vi "2dArrayTo1dArray.vi"(11 "2D Array":dbl[][](array[numeric])) -> (3 "1D Array":dbl[](array[numeric]))   [LabVIEW 2016]
doc: "Reshape the 2D array to 1D array."
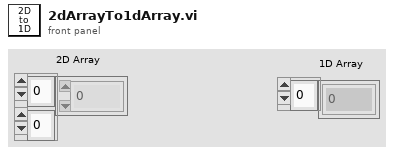
[diagram p1: front panel]
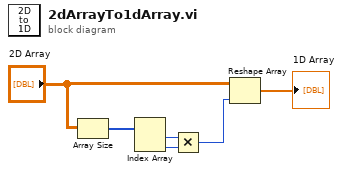
[diagram p0: block diagram]
diagram:
  n1 = Array Size(array="2D Array") -> (size(s)=w6:i32[])
  n2 = Index Array(array=w6) -> (element #1=w4:i32, element #2=w5:i32)  [unwired: 2 in]
  n3 = Multiply(x=w4, y=w5) -> (x*y=w2:i32)
  n4 = Reshape Array("2D Array", w2) -> (→"1D Array":dbl[])
